vi "get_absolute_class_path.vi"(4 "error in (no error)":errorcluster, 6 "Container State":T2, 7 "Display State In":T1={"configuration visible?"=TRUE, "label visible?"=TRUE, "settings visible?"=TRUE, "start path"=path ""}) -> (0 "error out":errorcluster, 2 "Value":path, 3 "Display State Out":T1={"configuration visible?"=TRUE, "label visible?"=TRUE, "settings visible?"=TRUE, "start path"=path ""})   [LabVIEW 2010, in "XComponentSpecification.xctl"]
uses:
  XComponentSpecification.xctl
  <vilib>/_xctls/Container State.ctl
  state.ctl
  data.ctl
  <vilib>/_xctls/XControlSupport.lvlib
panel:
  # "Replace the Value Indicator below with an Indicator of desired type.\nDo not remove this Indicator or the others from the connector pane. \nDo not change the connector pane pattern.\nThe Value Indicator should always be the second terminal from top on the output side in the connector pane."
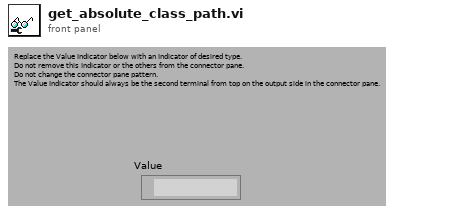
[diagram p1: front panel]
types:
  T1 = typedef "XComponentSpecification.xctl/state.ctl" = cluster{"configuration visible?":bool, "label visible?":bool, "settings visible?":bool, "start path":path}
  T2 = typedef "XControlSupport.lvlib/Container State.ctl" = cluster{"Indicator?":bool, "Run Mode?":bool, " Refnum":refnum<vi>}
  T3 = typedef "XComponentSpecification.xctl/data.ctl" = cluster{"class path":string, "configuration":string, "label":string, "settings name":string}
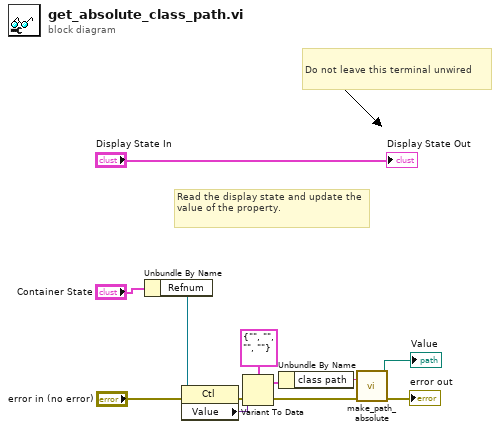
[diagram p0: block diagram]
diagram:
  # "Do not leave this terminal unwired"
  # "Read the display state and update the value of the property."
  n1 = Unbundle By Name("Container State") -> ("Refnum"=w11:refnum<vi>)
  n2 = property class="Ctl"(reference=w11, error in="error in (no error)") -> (error out=w8:errorcluster, "Value"=w9:variant)  [unwired: 1 out]
  n3 = Variant To Data(error in=w8, Variant=w9, type=T3 {"class path"="", "configuration"="", "label"="", "settings name"=""} ("component specification")) -> (error out=w7:errorcluster, data=w6:T3)
  n4 = Unbundle By Name(w6) -> ("class path"=w5:string)
  n5 = call "make_path_absolute.vi"("error in (no error)"=w7, "relative path"=w5) -> ("error out"=→"error out":errorcluster, "absolute path"=→"Value":path)  [unwired: 8 in]
  "Display State Out" <- "Display State In"
